vi "Error Fork Stacker.vi"(3 "Error Fork B":errorcluster, 4 "Error Fork A":errorcluster) -> (2 "Error Out":errorcluster)   [LabVIEW 2018, in "monoDrive.lvlib"]
uses:
  C:/Users/celit/Documents/GitHub/client/examples/labview/monoDrive.lvlib
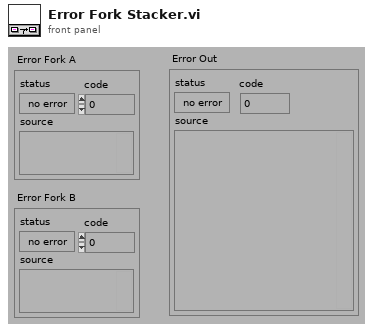
[diagram p1: front panel]
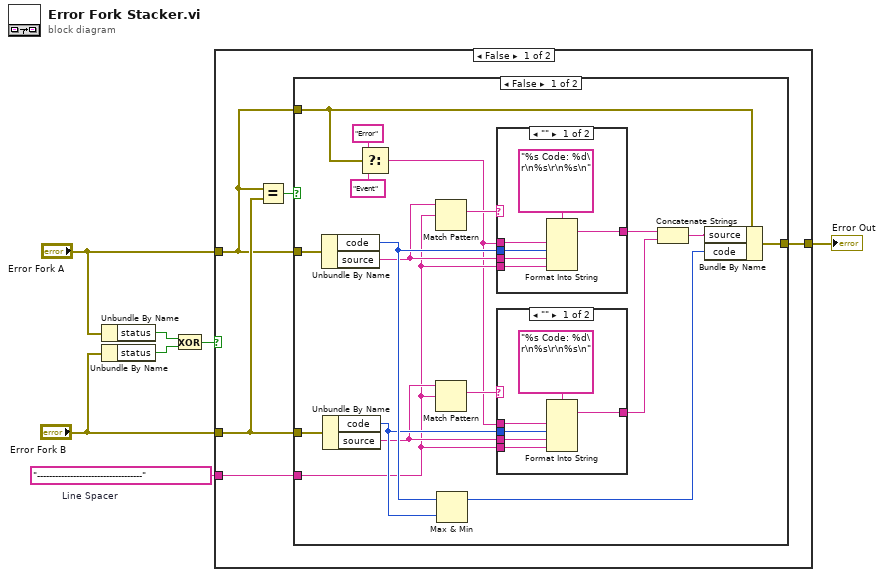
[diagram p0: block diagram]
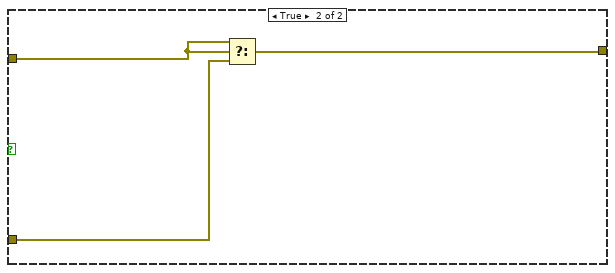
[diagram p5: hidden frame]
diagram:
  w4 = "-----------------------------------"  # Line Spacer
  n1 = Unbundle By Name("Error Fork A") -> ("status"=w3:bool)
  n2 = Unbundle By Name("Error Fork B") -> ("status"=w2:bool)
  n3 = Exclusive Or(1:w2, 2:w3) -> (0:w1:bool)
  n4 = case shown="False" w1 {
    tunnel: [w11 w48] -> w7
    tunnel: "Error Fork A" -> [w8 w47]
    tunnel: "Error Fork B" -> [w10 w46]
    tunnel: w4 -> [w9 _]
    frame False {
      n5 = Equal?(x=w8, y=w10) -> (x = y?=w12:bool)
      n6 = case shown="False" w12 {
        tunnel: w8 -> [w27 w45]
        tunnel: [w28 w45] -> w11
        tunnel: w10 -> [w29 _]
        tunnel: w8 -> [w14 _]
        tunnel: w9 -> [w17 _]
        frame False {
          n7 = Unbundle By Name(w27) -> ("code"=w24:i32, "source"=w19:string)
          n8 = Unbundle By Name(w29) -> ("code"=w23:i32, "source"=w18:string)
          n9 = Select(t="Error" ("source"), s=w14, f="Event" ("source")) -> (s? t:f=w16:string)
          n10 = Match Pattern(string=w19, regular expression=w17) -> (match substring=w21:string)  [unwired: 1 in, 3 out]
          n11 = Match Pattern(string=w18, regular expression=w17) -> (match substring=w20:string)  [unwired: 1 in, 3 out]
          n12 = Max & Min(x=w24, y=w23) -> (max(x,y)=w30:i32)  [unwired: 1 out]
          n13 = case shown="\"\"" w21 {
            tunnel: [w43 w44] -> w26
            tunnel: w24 -> [w42 _]
            tunnel: w19 -> [w40 w44]
            tunnel: w17 -> [w39 _]
            tunnel: w16 -> [w38 _]
            frame "" {
              n14 = Format Into String(format string="%s Code: %d\r\n%s\r\n%s\n" ("source"), w38, w42, w40, w39) -> (resulting string=w43:string)  [unwired: 2 in, 1 out]
            }
            frame Default {
            }
          }
          n15 = case shown="\"\"" w20 {
            tunnel: [w36 w37] -> w22
            tunnel: w23 -> [w35 _]
            tunnel: w18 -> [w33 w37]
            tunnel: w17 -> [w32 _]
            tunnel: w16 -> [w31 _]
            frame "" {
              n16 = Format Into String(format string="%s Code: %d\r\n%s\r\n%s\n" ("source"), w31, w35, w33, w32) -> (resulting string=w36:string)  [unwired: 2 in, 1 out]
            }
            frame Default {
            }
          }
          n17 = Concatenate Strings(w26, w22) -> (w25:string)
          n18 = Bundle By Name(cluster=w14, "source"=w25, "code"=w30) -> (w28:errorcluster)
        }
        frame True {
        }
      }
    }
    frame True {
      n19 = Select(t=w47, s=w47, f=w46) -> (s? t:f=w48:errorcluster)
    }
  }
  "Error Out" <- w7
